vi "WriteBuffer.vi"(5 "Pointer and BufferSize":u64[](array[numeric]), 7 "element":i16, 9 "Buffer size":i32, 11 "error in (no error)":errorcluster) -> (6 "Pointer and BufferSize Out":u64[](array[numeric]), 15 "error out":errorcluster)   [LabVIEW 2010]
uses:
  <vilib>/Utility/error.llb/DialogType.ctl
panel:
  in  "type of dialog (OK msg:1)":T1=4 items=["no dialog", "OK message", "continue or stop message", "OK message + warnings", "continue/stop + warnings"]
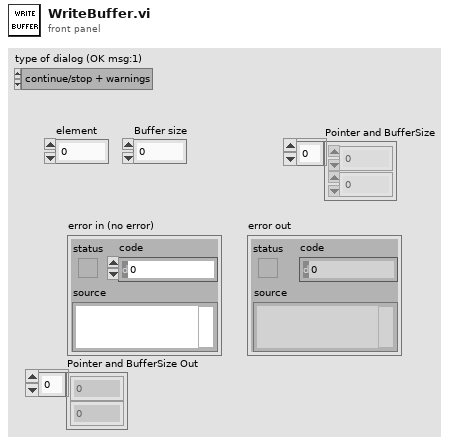
[diagram p1: front panel]
types:
  T1 = typedef "DialogType.ctl" = u16
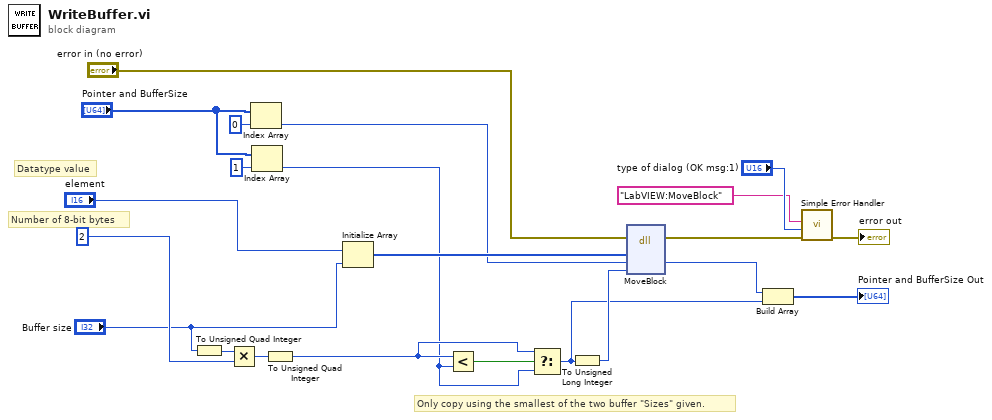
[diagram p0: block diagram]
diagram:
  # "Number of 8-bit bytes"
  # "Datatype value"
  # "Only copy using the smallest of the two buffer \"Sizes\" given."
  n1 = To Unsigned Quad Integer(1:"Buffer size") -> (0:w12:u64)
  n2 = Multiply(x=w12, y=u64 2) -> (x*y=w18:u64)
  n3 = Index Array(array="Pointer and BufferSize", index=0) -> (element=w5:u64)
  n4 = Index Array(array="Pointer and BufferSize", index=1) -> (element=w10:u64)
  n5 = To Unsigned Quad Integer(1:w18) -> (0:w15:u64)
  n6 = Initialize Array("element", "Buffer size") -> (w16:i16[])
  n7 = Less?(x=w15, y=w10) -> (x < y?=w14:bool)
  n8 = Select(t=w15, s=w14, f=w10) -> (s? t:f=w1:u64)
  n9 = To Unsigned Long Integer(number=w1) -> (unsigned 32bit integer=w2:u32)
  n10 = dll-call lib="LabVIEW" fn="MoveBlock"(error in="error in (no error)", "Source"=w16, "Destination_Pointer"=w5, "Size"=w2) -> (error out=w7:errorcluster, "Destination_Pointer"=w3:u64)  [unwired: 5 in, 1 out]
  n11 = Build Array(w3, w1) -> (→"Pointer and BufferSize Out":u64[])
  n12 = call <vilib>:"Simple Error Handler.vi"("error source (\" \")"="LabVIEW:MoveBlock", "type of dialog (OK msg:1)"="type of dialog (OK msg:1)", "error in (no error)"=w7) -> ("error out"=→"error out":errorcluster)  [unwired: 2 in, 4 out]
